vi "4Pi 4Pi Modes - Vectorise Coefficients.vi"(0 "Coefficients In":cluster{"Mode":string, "Amplitude":dbl}[](array[cluster])) -> (4 "Coefficients Out":cluster{"Amplitudes":dbl[], "Modes":string[]})   [LabVIEW 2016]
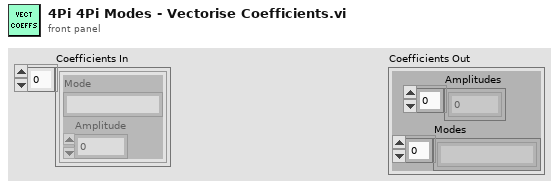
[diagram p1: front panel]
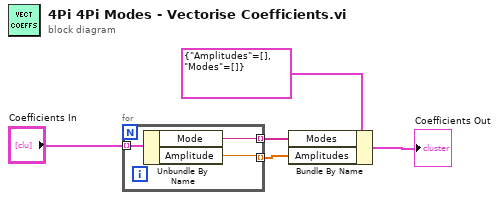
[diagram p0: block diagram]
diagram:
  n1 = for {
    tunnel: "Coefficients In" -> [w8] mode=indexing
    tunnel: [w7] -> w4 mode=indexing
    tunnel: [w6] -> w3 mode=indexing
    n2 = Unbundle By Name(w8) -> ("Mode"=w7:string, "Amplitude"=w6:dbl)
  }
  n3 = Bundle By Name(cluster=cluster{"Amplitudes":dbl[], "Modes":string[]} {"Amplitudes"=[], "Modes"=[]}, "Modes"=w4, "Amplitudes"=w3) -> (→"Coefficients Out":cluster{"Amplitudes":dbl[], "Modes":string[]})
